vi "CC_G2_v2_sub.vi"(2 "skip n":i16, 3 "Macros2":i32[](array[numeric])=array[45080 elements], 4 "Macros1":i32[](array[numeric])=array[45080 elements]) -> (0 "Tau Values":dbl[](array[numeric]) format="%.6f", 1 "G2 vals":dbl[](array[numeric]) format="%.2f")   [LabVIEW 2009]
panel:
  in  "Numeric":i32=1000
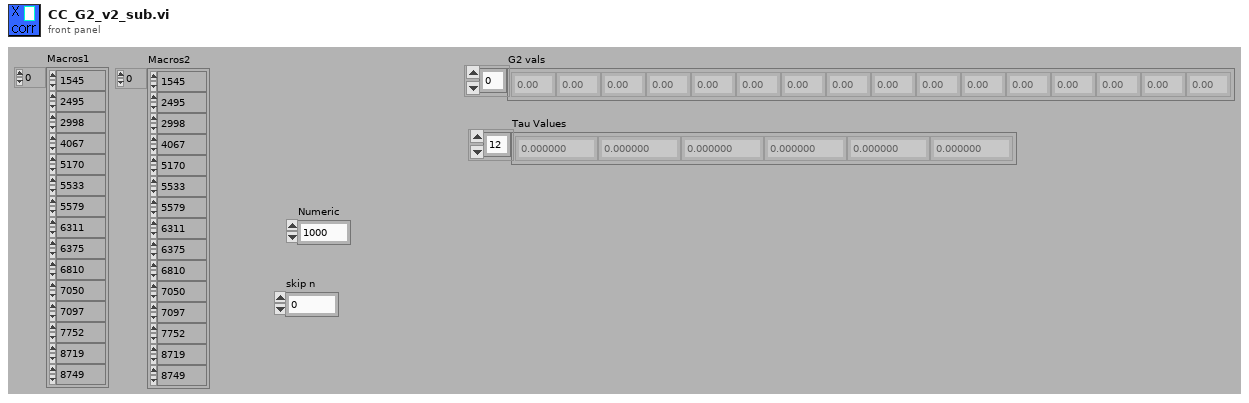
[diagram p1: front panel]
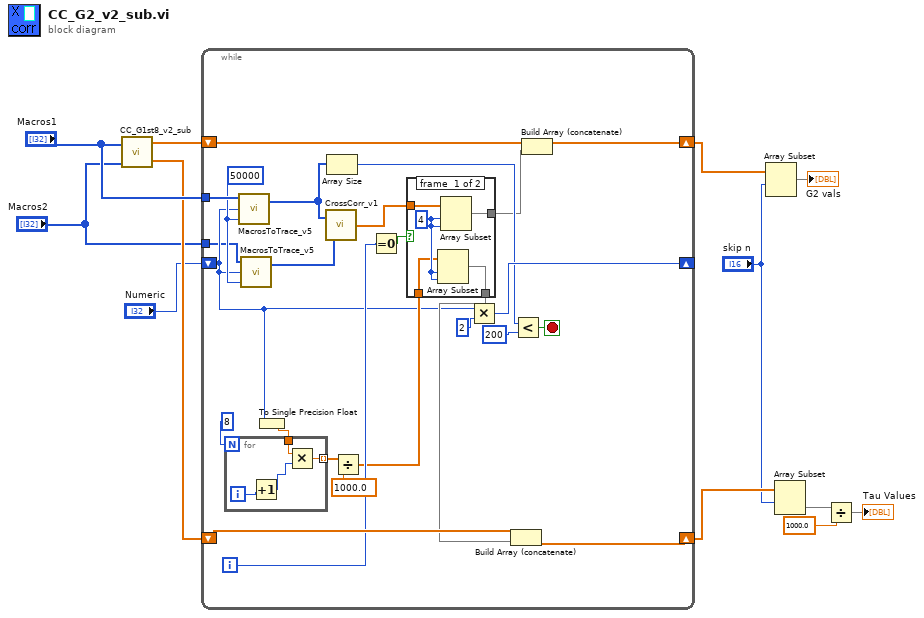
[diagram p0: block diagram]
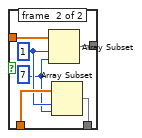
[diagram p2: hidden frame]
diagram:
  n1 = call "CC_G1st8_v2_sub.vi"("macros2"="Macros2", "macros1"="Macros1") -> ("Taus"=w11:dbl[], "G1st8"=w10:dbl[])
  n2 = while {
    shift-right: [w36] -> _
    shift-left: "Numeric" -> [w17]
    shift-right: [w28] -> w5
    shift-left: w10 -> [w32]
    shift-right: [w31] -> w3
    shift-left: w11 -> [w30]
    tunnel: "Macros1" -> [w24]
    tunnel: "Macros2" -> [w16]
    i -> [w23]
    stop <- w26 stop-if-true
    w18 = 50000 ("clocktimePS")
    n3 = call "MacrosToTrace_v5.vi"("clocktimePS"=w18, "BintimeNS"=w17, "Macros"=w24) -> ("Trace"=w13:i32[])  [unwired: 1 out]
    n4 = call "MacrosToTrace_v5.vi"("clocktimePS"=w18, "BintimeNS"=w17, "Macros"=w16) -> ("Trace"=w15:i32[])  [unwired: 1 out]
    n5 = To Single Precision Float(number=w17) -> (single precision float=w29:sgl)
    n6 = for {
      N: 8 -> [_]
      tunnel: [w49] -> w35 mode=indexing
      tunnel: w29 -> [w51]
      i -> [w52]
      n7 = Increment(x=w52) -> (x+1=w50:i32)
      n8 = Multiply(x=w51, y=w50) -> (x*y=w49:sgl)
    }
    n9 = call "CrossCorr_v1.vi"("Trace2"=w15, "Trace1"=w13) -> ("G1-G8"=w14:dbl[])
    n10 = Array Size(array=w13) -> (size(s)=w25:i32)
    n11 = Divide(x=w35, y=sgl 1000.0) -> (x/y=w20:sgl[])
    n12 = Equal To 0?(x=w23) -> (x = 0?=w22:bool)
    n13 = case shown="True" w22 {
      tunnel: w14 -> [w42 w48]
      tunnel: [w41 w47] -> w21
      tunnel: w20 -> [w39 w46]
      tunnel: [w38 w45] -> w19
      frame #0 {
        w40 = 4 ("index")
        n14 = Array Subset(array=w39, index=w40, length=w40) -> (w38:sgl[])
        n15 = Array Subset(array=w42, index=w40, length=w40) -> (w41:dbl[])
      }
      frame #1 {
        w43 = 7 ("index")
        w44 = 1 ("index")
        n16 = Array Subset(array=w48, index=w44, length=w43) -> (w47:dbl[])
        n17 = Array Subset(array=w46, index=w44, length=w43) -> (w45:sgl[])
      }
    }
    n18 = Multiply(x=w17, y=2) -> (x*y=w36:i32)
    n19 = Build Array (concatenate)(w30, w19) -> (w31:dbl[])
    n20 = Less?(x=w25, y=200) -> (x < y?=w26:bool)
    n21 = Build Array (concatenate)(w32, w21) -> (w28:dbl[])
  }
  n22 = Array Subset(array=w5, index="skip n") -> (→"G2 vals":dbl[])  [unwired: 1 in]
  n23 = Array Subset(array=w3, index="skip n") -> (w2:dbl[])  [unwired: 1 in]
  n24 = Divide(x=w2, y=1000.0) -> (x/y=→"Tau Values":dbl[])
